vi "AUTOFLIM_MoveMirror.vi"(11 "Numeric":i16) -> ()   [LabVIEW 2016]
panel:
  in  "MG17Motor":refnum<k7>(container)
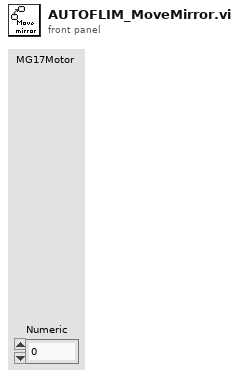
[diagram p1: front panel]
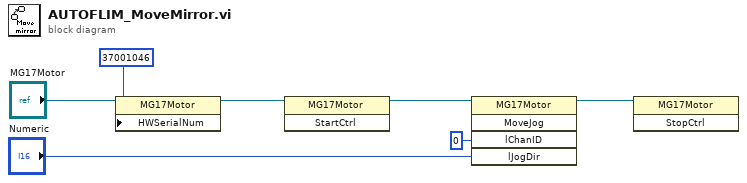
[diagram p0: block diagram]
diagram:
  n1 = property class="MG17Motor"(reference="MG17Motor", "HWSerialNum"=37001046) -> (reference out=w5:refnum<k7>)  [unwired: 1 in, 1 out]
  n2 = invoke class="MG17Motor" method="StartCtrl"(reference=w5) -> (reference out=w2:refnum<k7>)  [unwired: 2 in, 2 out]
  n3 = invoke class="MG17Motor" method="MoveJog"(reference=w2, "lChanID"=0, "lJogDir"="Numeric") -> (reference out=w1:refnum<k7>)  [unwired: 2 in, 4 out]
  n4 = invoke class="MG17Motor" method="StopCtrl"(reference=w1) -> ()  [unwired: 2 in, 3 out]
